vi "Construct Terminal Value Binding.vi"(10 "Ctl Refnum":refnum<vi>, 11 "TerminalValueBinding In":refnum<class "TerminalValueBinding.lvclass">) -> (0 "error out":errorcluster, 3 "TerminalValueBinding Out":refnum<class "TerminalValueBinding.lvclass">)   [LabVIEW 2018, in "MVA Framework.lvlib" / "TerminalValueBinding.lvclass"]
doc: "构建终端值绑定"
uses:
  TerminalValueBinding.lvclass
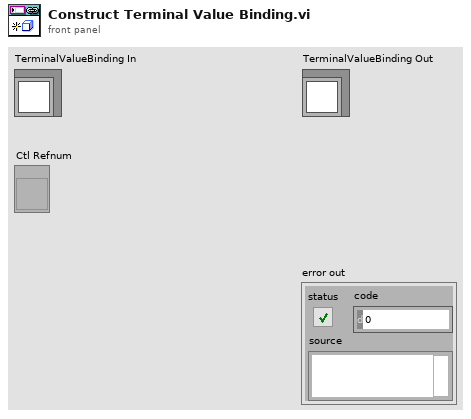
[diagram p1: front panel]
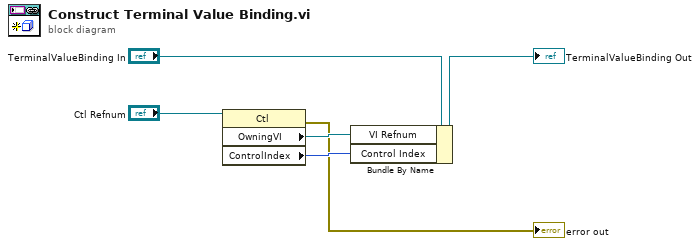
[diagram p0: block diagram]
diagram:
  n1 = property class="Ctl"(reference="Ctl Refnum") -> (error out=→"error out":errorcluster, "OwningVI"=w4:refnum<vi>, "ControlIndex"=w3:i32)  [unwired: 1 in, 1 out]
  n2 = Bundle By Name(cluster="TerminalValueBinding In", "VI Refnum"=w4, "Control Index"=w3) -> (→"TerminalValueBinding Out":refnum<class "TerminalValueBinding.lvclass">)
